vi "REMOVE SALE ITEMS.vi"(11 "REFERENCES":T1) -> ()   [LabVIEW 2019]
uses:
  Controls/References Cluster.ctl
  <vilib>/userDefined/High Color/IMAQdx.ctl
  Controls/Custom Calendar/Custom Calendar.xctl
types:
  T1 = typedef "References Cluster.ctl" = cluster{"MAIN PAGES":refnum<vi>, "ADD/EDIT ITEM REFERENCES":cluster{"Identifier":refnum<vi>, "BYU ICN #":refnum<vi>, "Item Description":refnum<vi>, "Comments":refnum<vi>, "Checked Out Date":refnum<vi>, "Due Date":refnum<vi>, "Check Out Location":refnum<vi>, "Reminder Count":refnum<vi>, "Most Recent Reminder Date":refnum<vi>, "BYU ID #":refnum<vi>, "Building/Room":refnum<vi>, "Location in Room":refnum<vi>, "Manual":refnum<vi>, "Manufacturer":refnum<vi>, "Model #":refnum<vi>, "Serial #":refnum<vi>, "Date Acquired":refnum<vi>, "ADD/EDIT ITEM LABEL":refnum<vi>, "ARCHIVE ITEM":refnum<vi>, "Archive Item Inputs":refnum<vi>, "Reminder Notes":refnum<vi>, "DUPLICATE ITEM":refnum<vi>}, "ADD/EDIT USER REFERENCES":cluster{"BYU ID # (##-###-####)":refnum<vi>, "First Name":refnum<vi>, "Last Name":refnum<vi>, "Phone Number (###-###-####)":refnum<vi>, "Email":refnum<vi>, "Department":refnum<vi>, "Graduation Status":refnum<vi>, "Anticipated Graduation Year":refnum<vi>, "Credit Score":refnum<vi>, "Date Added":refnum<vi>, "Graduation Clearance Date":refnum<vi>, "Picture File Name":refnum<vi>, "ADD/EDIT USER LABEL":refnum<vi>, "Department Map":refnum<vi>, "Status Map":refnum<vi>, "Anticipated Graduation Year Map":refnum<vi>, "User Agreement":refnum<vi>, "User Comments":refnum<vi>, "Camera":refnum<vi>}, "RETURN ITEM REFERENCES":cluster{"Item or Person:":refnum<vi>, "Search Return Results":refnum<vi>, "What are you searching for?":refnum<vi>}, "SEARCH DATABASE REFERENCES":cluster{"What to Search For:":refnum<vi>, "Where to Search":refnum<vi>, "Column to Search In":refnum<vi>, "Column to Sort By":refnum<vi>, "Search Database Results":refnum<vi>, "Inventory Column Selector":refnum<vi>, "User Column Selector":refnum<vi>, "Inventory Archive Column Selector":refnum<vi>, "User Archive Column Selector":refnum<vi>, "Sales Tracking Column Selector":refnum<vi>, "Checked In Archive Column Selector":refnum<vi>, "Restore User":refnum<vi>, "Date Range":refnum<vi>, "Dates Less Than":refnum<vi>, "Dates Greater Than":refnum<vi>, "Search Print Receipt":refnum<vi>, "Edit Sale Description":refnum<vi>}, "USER ITEMS REFERENCES":cluster{"USER'S INFORMATION":refnum<vi>, "User's Checked Out Items":refnum<vi>, "User Info Comments":refnum<vi>, "SEE USER INFO COMMENTS":refnum<vi>}, "EDIT ITEMS REFERENCES":cluster{"New Check Out Location":refnum<vi>, "Items to Edit":refnum<vi>, "Edit Items Due Date":refnum<vi>, "New Reminder Notes":refnum<vi>, "New Item Description":refnum<vi>}, "CHECK OUT ITEMS REFERENCES":cluster{"Enter Item:":refnum<vi>, "Check Out Items Due Date":refnum<vi>, "Check Out Location":refnum<vi>, "Items to be Checked Out":refnum<vi>, "Possible Items":refnum<vi>, "Altered Item Description":refnum<vi>}, "TRANSFER ITEMS REFERENCES":cluster{"Search Parameter":refnum<vi>, "What to Match":refnum<vi>, "Matching Individuals":refnum<vi>, "Items to be Transferred":refnum<vi>}, "SETTINGS REFERENCES":cluster{"PSC Database Settings":refnum<vi>, "PSC Sales Item Spreadsheet":refnum<vi>}, "PSC SALES REFERENCES":cluster{"BYU ID CARD #":refnum<vi>, "Sale Description":refnum<vi>, "Scan or Enter Item Name":refnum<vi>, "Items to be Sold":refnum<vi>, "Grand Total":refnum<vi>, "Item List":refnum<vi>}}
  T2 = cluster{"BYU ID CARD #":refnum<vi>, "Sale Description":refnum<vi>, "Scan or Enter Item Name":refnum<vi>, "Items to be Sold":refnum<vi>, "Grand Total":refnum<vi>, "Item List":refnum<vi>}
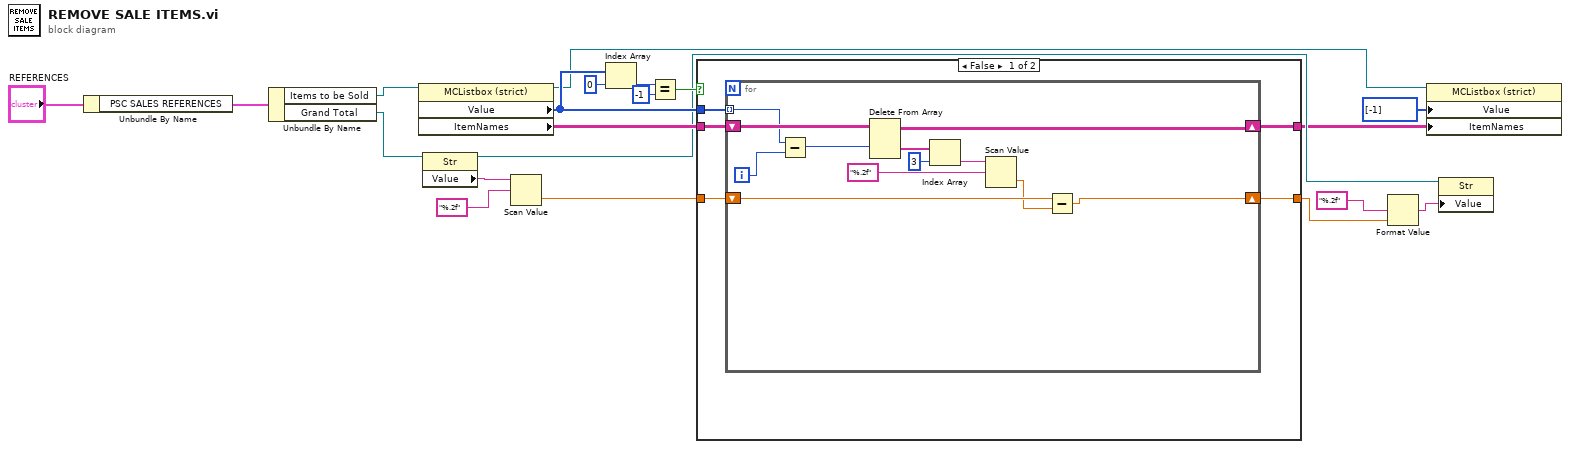
[diagram p0: block diagram]
diagram:
  n1 = Unbundle By Name("REFERENCES") -> ("PSC SALES REFERENCES"=w19:T2)
  n2 = Unbundle By Name(w19) -> ("Items to be Sold"=w18:refnum<vi>, "Grand Total"=w17:refnum<vi>)
  n3 = property class="MCListbox (strict)"(reference=w18) -> (reference out=w6:refnum<vi>, "Value"=w8:i32[], "ItemNames"=w9:string[][])  [unwired: 1 in, 1 out]
  n4 = property class="Str"(reference=w17) -> (reference out=w7:refnum<vi>, "Value"=w16:string)  [unwired: 1 in, 1 out]
  n5 = Scan Value(string=w16, format string="%.2f") -> (value=w10:dbl)  [unwired: 1 in, 1 out]
  n6 = Index Array(array=w8, index=0) -> (element=w13:i32)
  n7 = Equal?(x=w13, y=-1) -> (x = y?=w11:bool)
  n8 = case shown="False" w11 {
    tunnel: w10 -> [w23 w38]
    tunnel: w9 -> [w25 w39]
    tunnel: w8 -> [w24 _]
    tunnel: [w22 w39] -> w4
    tunnel: [w21 w38] -> w3
    frame False {
      n9 = for {
        tunnel: w24 -> [w36] mode=indexing
        shift-right: [w33] -> w22
        shift-left: w25 -> [w37]
        shift-right: [w26] -> w21
        shift-left: w23 -> [w28]
        i -> [w35]
        n10 = Subtract(x=w36, y=w35) -> (x-y=w34:i32)
        n11 = Delete From Array(array=w37, index (row)=w34) -> (deleted portion=w32:string[], array with subset deleted=w33:string[][])  [unwired: 2 in]
        n12 = Index Array(array=w32, index=3) -> (element=w30:string)
        n13 = Scan Value(string=w30, format string="%.2f") -> (value=w27:dbl)  [unwired: 1 in, 1 out]
        n14 = Subtract(x=w28, y=w27) -> (x-y=w26:dbl)
      }
    }
    frame True {
    }
  }
  n15 = Format Value(format string="%.2f", value (0)=w3) -> (output string=w1:string)  [unwired: 1 in]
  n16 = property class="MCListbox (strict)"(reference=w6, "Value"=i32[] [-1], "ItemNames"=w4) -> ()  [unwired: 1 in, 2 out]
  n17 = property class="Str"(reference=w7, "Value"=w1) -> ()  [unwired: 1 in, 2 out]
